vi "8Bit RAM chip.vi"(1 "Clock":bool, 2 "Address":bool[](array[boolean])=[FALSE, FALSE, FALSE, FALSE, FALSE, FALSE, FALSE, FALSE, FALSE, FALSE, FALSE, FALSE, FALSE, FALSE, FALSE, FALSE], 3 "Data In":bool[](array[boolean])=[FALSE, FALSE, FALSE, FALSE, FALSE, FALSE, FALSE, FALSE, FALSE, FALSE, FALSE, FALSE, FALSE, FALSE, FALSE, FALSE], 4 "Hold":bool) -> (0 "Reg Out 1":bool[](array[boolean]))   [LabVIEW 2012]
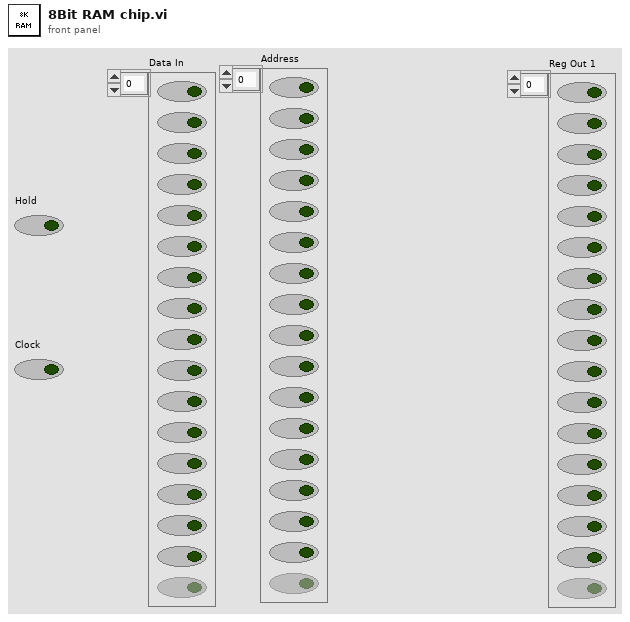
[diagram p1: front panel]
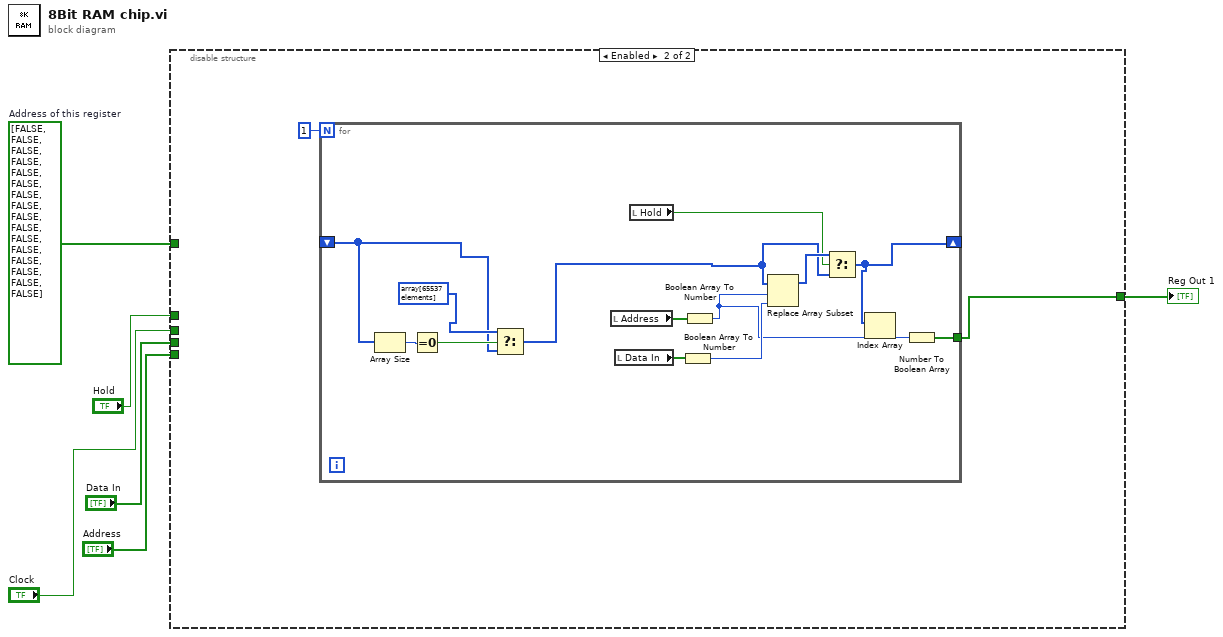
[diagram p0: block diagram]
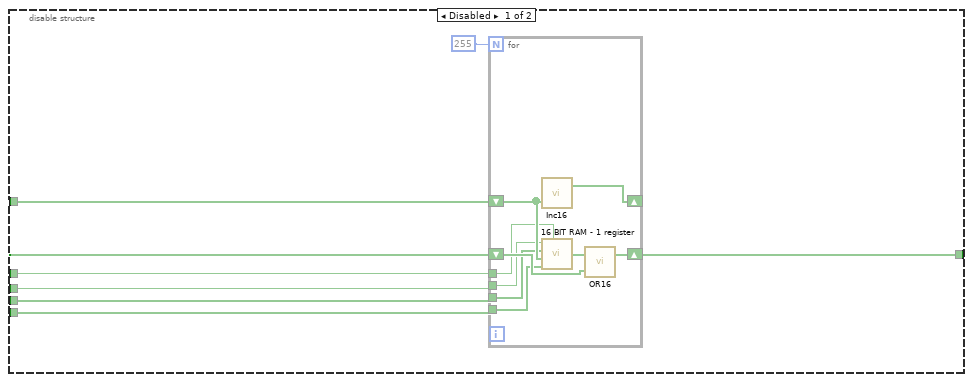
[diagram p2: hidden frame]
diagram:
  w6 = bool[] [FALSE, FALSE, FALSE, FALSE, FALSE, FALSE, FALSE, FALSE, FALSE, FALSE, FALSE, FALSE, FALSE, FALSE, FALSE, FALSE]  # Address of this register
  n1 = disable-structure shown="Enabled" {
    disable-tunnel: w6 -> [w13 _]
    disable-tunnel: [w12 w23] -> w5
    disable-tunnel: "Clock" -> [w10 _]
    disable-tunnel: "Address" -> [w9 _]
    disable-tunnel: "Data In" -> [w8 _]
    disable-tunnel: "Hold" -> [w7 _]
    frame Disabled {
      n2 = for {
        N: u16 255 -> [_]
        shift-right: [w21] -> _
        shift-left: w13 -> [w22]
        shift-right: [w18] -> w12
        shift-left: w13 -> [w20]
        tunnel: w10 -> [w17]
        tunnel: w9 -> [w16]
        tunnel: w7 -> [w14]
        tunnel: w8 -> [w15]
        n3 = call "Inc16.vi"("A"=w22) -> ("S"=w21:bool[])  [unwired: 1 in, 1 out]
        n4 = call "16 BIT RAM - 1 register.vi"("Hold"=w14, "Address"=w16, "Address of this register"=w22, "Data In"=w15, "Clock"=w17) -> ("z"=w19:bool[])  [unwired: 1 in]
        n5 = call "OR16.vi"("B"=w20, "A"=w19) -> ("z"=w18:bool[])  [unwired: 1 out]
      }
    }
    frame Enabled {
      n6 = for {
        N: 1 -> [_]
        shift-right: [w33] -> _
        shift-left: _ -> [w26]
        tunnel: [w30] -> w23
        n7 = Array Size(array=w26) -> (size(s)=w29:i32)
        n8 = Equal To 0?(x=w29) -> (x = 0?=w28:bool)
        n9 = Select(t=u16[] array[65537 elements], s=w28, f=w26) -> (s? t:f=w25:u16[])
        n10 = local read "Address"() -> (w38:bool[])
        n11 = local read "Data In"() -> (w37:bool[])
        n12 = local read "Hold"() -> (w34:bool)
        n13 = Boolean Array To Number(Boolean array=w37) -> (number=w36:u32)
        n14 = Boolean Array To Number(Boolean array=w38) -> (number=w32:u32)
        n15 = Replace Array Subset(array=w25, new element=w36, index=w32) -> (w35:u16[])
        n16 = Select(t=w35, s=w34, f=w25) -> (s? t:f=w33:u16[])
        n17 = Index Array(array=w33, index=w32) -> (element=w31:u16)
        n18 = Number To Boolean Array(number=w31) -> (Boolean array=w30:bool[])
      }
    }
  }
  "Reg Out 1" <- w5
